vi "AutoCorrelation PtByPt (obs 85).vi"(2 "initialize":bool, 3 "sample length x":i32=100, 5 "x":dbl format="%0.2f") -> (0 "error":i32, 1 "Rxx":dbl[](array[numeric]))   [LabVIEW 2020, in "NI_PtbyPt.lvlib"]
doc: "Computes the autocorrelation of the set of input data points specified by <B>sample length x</B>."
uses:
  <vilib>/ptbypt/NI_PtbyPt.lvlib
panel:
  # "This VI is obsolete !!!\nYou should replace this VI in your diagram with the AutoCorrelation PtByPt VI.\n\nNOTE: Please be aware of that the new AutoCorrelation PtByPt VI is set to \n           reentrant."
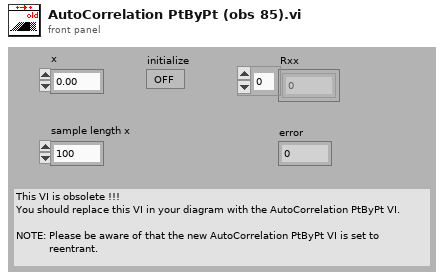
[diagram p1: front panel]
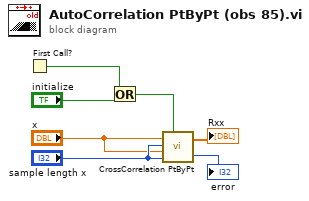
[diagram p0: block diagram]
diagram:
  n1 = First Call?() -> (First Call?: T/F=w2:bool)
  n2 = Or(x=w2, y="initialize") -> (x .or. y?=w1:bool)
  n3 = call <vilib>:"CrossCorrelation PtByPt.vi"("x"="x", "sample length x"="sample length x", "y"="x", "sample length y"="sample length x", "initialize"=w1) -> ("Rxy"=→"Rxx":dbl[], "error"=→"error":i32)
